vi "CH_LM DFM Change Directory.vi"(0 "Meter Index":i32, 2 "Directory Name (\"\")":string, 5 "error in (no error)":errorcluster, 7 "Timeout / ms (3000)":i32=3000, 8 "Action (query)":bool, 9 "Lock Timeout / ms (1000)":i32=1000) -> (11 "Lock timed out":bool, 14 "Meter Index":i32, 16 "Woring Directory":string, 19 "error out":errorcluster)   [LabVIEW 2012, in "CH_LM.lvlib"]
doc: "This command will set/query the current working directory.\n\n<B>Attention:</B> An attempt to set the current working directory to a non-existent directory will raise error 200. The query will get the quoted current working directory. The current working directory will be the root directory of the internal data storage directory tree after a power off/on cycle."
uses:
  CH_LM.lvlib
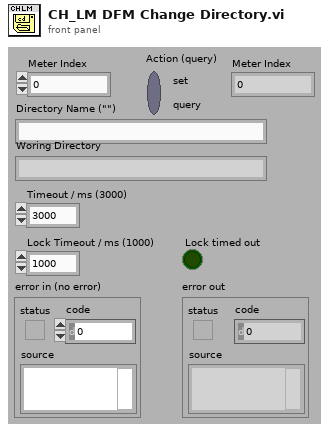
[diagram p1: front panel]
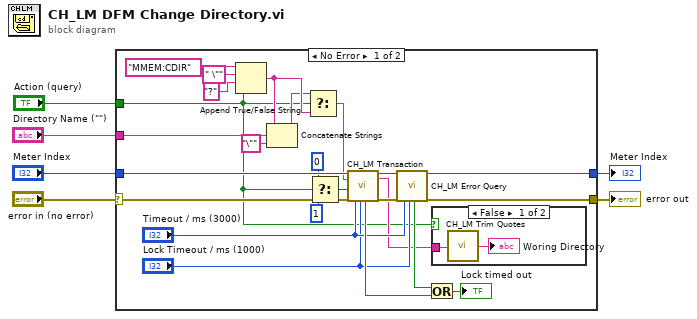
[diagram p0: block diagram]
diagram:
  n1 = case shown="No Error" "error in (no error)" {
    selector: "error in (no error)" -> [w30 w34]
    tunnel: [w27 w34] -> w6
    tunnel: "Meter Index" -> [w29 w33]
    tunnel: [w28 w33] -> w3
    tunnel: "Directory Name (\"\")" -> [w26 _]
    tunnel: "Action (query)" -> [w7 _]
    frame No Error {
      n2 = Append True/False String(1:w7, 2:"?", 3:" \"" ("true string"), 4:"MMEM:CDIR" ("Command String")) -> (0:w11:string)
      n3 = Concatenate Strings(w11, w26, "\"" ("string")) -> (w10:string)
      n4 = Select(t=w10, s=w7, f=w11) -> (s? t:f=w9:string)
      n5 = Select(t=0, s=w7, f=1 ("t")) -> (s? t:f=w14:i32)
      n6 = call "CH_LM Transaction.vi"("Meter Index"=w29, "Command String"=w9, "NofStrings (-1:all)"=w14, "error in (no error)"=w30, "Timeout / ms (3000)"="Timeout / ms (3000)", "Lock Timeout / ms (1000)"="Lock Timeout / ms (1000)") -> ("Lock timed out"=w22:bool, "Meter Index"=w25:i32, "Response"=w8:string, "error out"=w24:errorcluster)  [unwired: 10 out]
      n7 = call "CH_LM Error Query.vi"("Meter Index"=w25, "error in (no error)"=w24, "Timeout / ms (3000)"="Timeout / ms (3000)", "Lock Timeout / ms (1000)"="Lock Timeout / ms (1000)") -> ("Lock timed out"=w23:bool, "Meter Index"=w28:i32, "error out"=w27:errorcluster)  [unwired: 13 out]
      n8 = Or(x=w23, y=w22) -> (x .or. y?=→"Lock timed out":bool)
      n9 = case shown="False" w7 {
        tunnel: w8 -> [w32 _]
        frame False {
          n10 = call "CH_LM Trim Quotes.vi"("string"=w32) -> ("trimmed string"=→"Woring Directory":string)  [unwired: 1 in]
        }
        frame True {
        }
      }
    }
    frame Error {
    }
  }
  "error out" <- w6
  "Meter Index" <- w3
